vi "获取节点值（非属性）.vi"(11 "Xml Node":string) -> (3 "Xml Node Value":string)   [LabVIEW 2017]
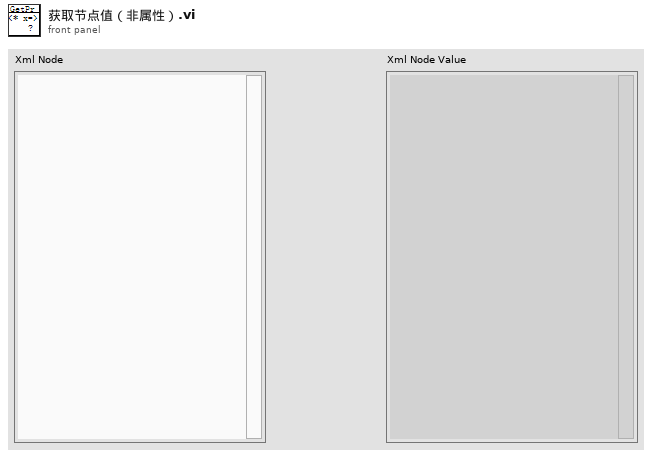
[diagram p1: front panel]
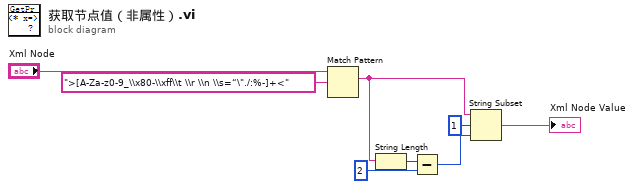
[diagram p0: block diagram]
diagram:
  n1 = Match Pattern(string="Xml Node", regular expression=">[A-Za-z0-9_\\x80-\\xff\\t \\r \\n \\s=“\"./:%-]+<" ("搜索字符串/字符(-)")) -> (match substring=w5:string)  [unwired: 1 in, 3 out]
  n2 = String Length(string=w5) -> (length=w4:i32)
  n3 = Subtract(x=w4, y=2) -> (x-y=w2:i32)
  n4 = String Subset(string=w5, offset (0)=1 ("偏移量(0)"), length (rest)=w2) -> (substring=→"Xml Node Value":string)
